vi "blinkLED.vi"   [LabVIEW 2015]
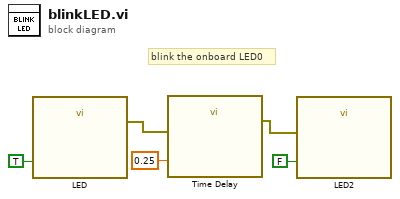
[diagram p0: block diagram]
diagram:
  # "blink the onboard LED0"
  n1 = call "LED"("LED0"=TRUE) -> ("error out"=w5:errorcluster)  [unwired: 26 in]
  n2 = call "Time Delay"("error in (no error)"=w5, "Delay Time (s)"=0.25) -> ("error out"=w4:errorcluster)  [unwired: 9 in]
  n3 = call "LED2"("LED0"=FALSE, "error in (no error)"=w4) -> ()  [unwired: 25 in, 1 out]
